vi "main.vi"() -> ()   [LabVIEW 2025]
uses:
  <vilib>/Handler Framework/CmdQueue/Enqueue Single.vi
  Classes/data log/data log.lvclass
  Classes/hardware/hardware.lvclass
  <vilib>/Handler Framework/Handler Framework.lvlib
panel:
  out "CMD Error":errorcluster
  out "x-y":dbl
  out "Waveform Chart":dbl(graph)
  out "Last Updated:":timestamp
  out "error out":errorcluster
  in  "save data":bool
  in  "Frequncy [Hz]":u16(slide)=1 max=10 step=1 scale=0.0..10.0
  in  "Reference Temperature [°F]":dbl(slide)=65.0 min=65.0 max=750.0 scale=0.0..500.0
  out "Temperatures:":dbl[](array[numeric]) format="%.1g"
  out "Duty Cycles:":dbl[](array[numeric]) format="%.1g"
  out "Relay Duty Cycle":T1(graph)
  out "Temperatures":T2(graph)
  in  "heat":bool
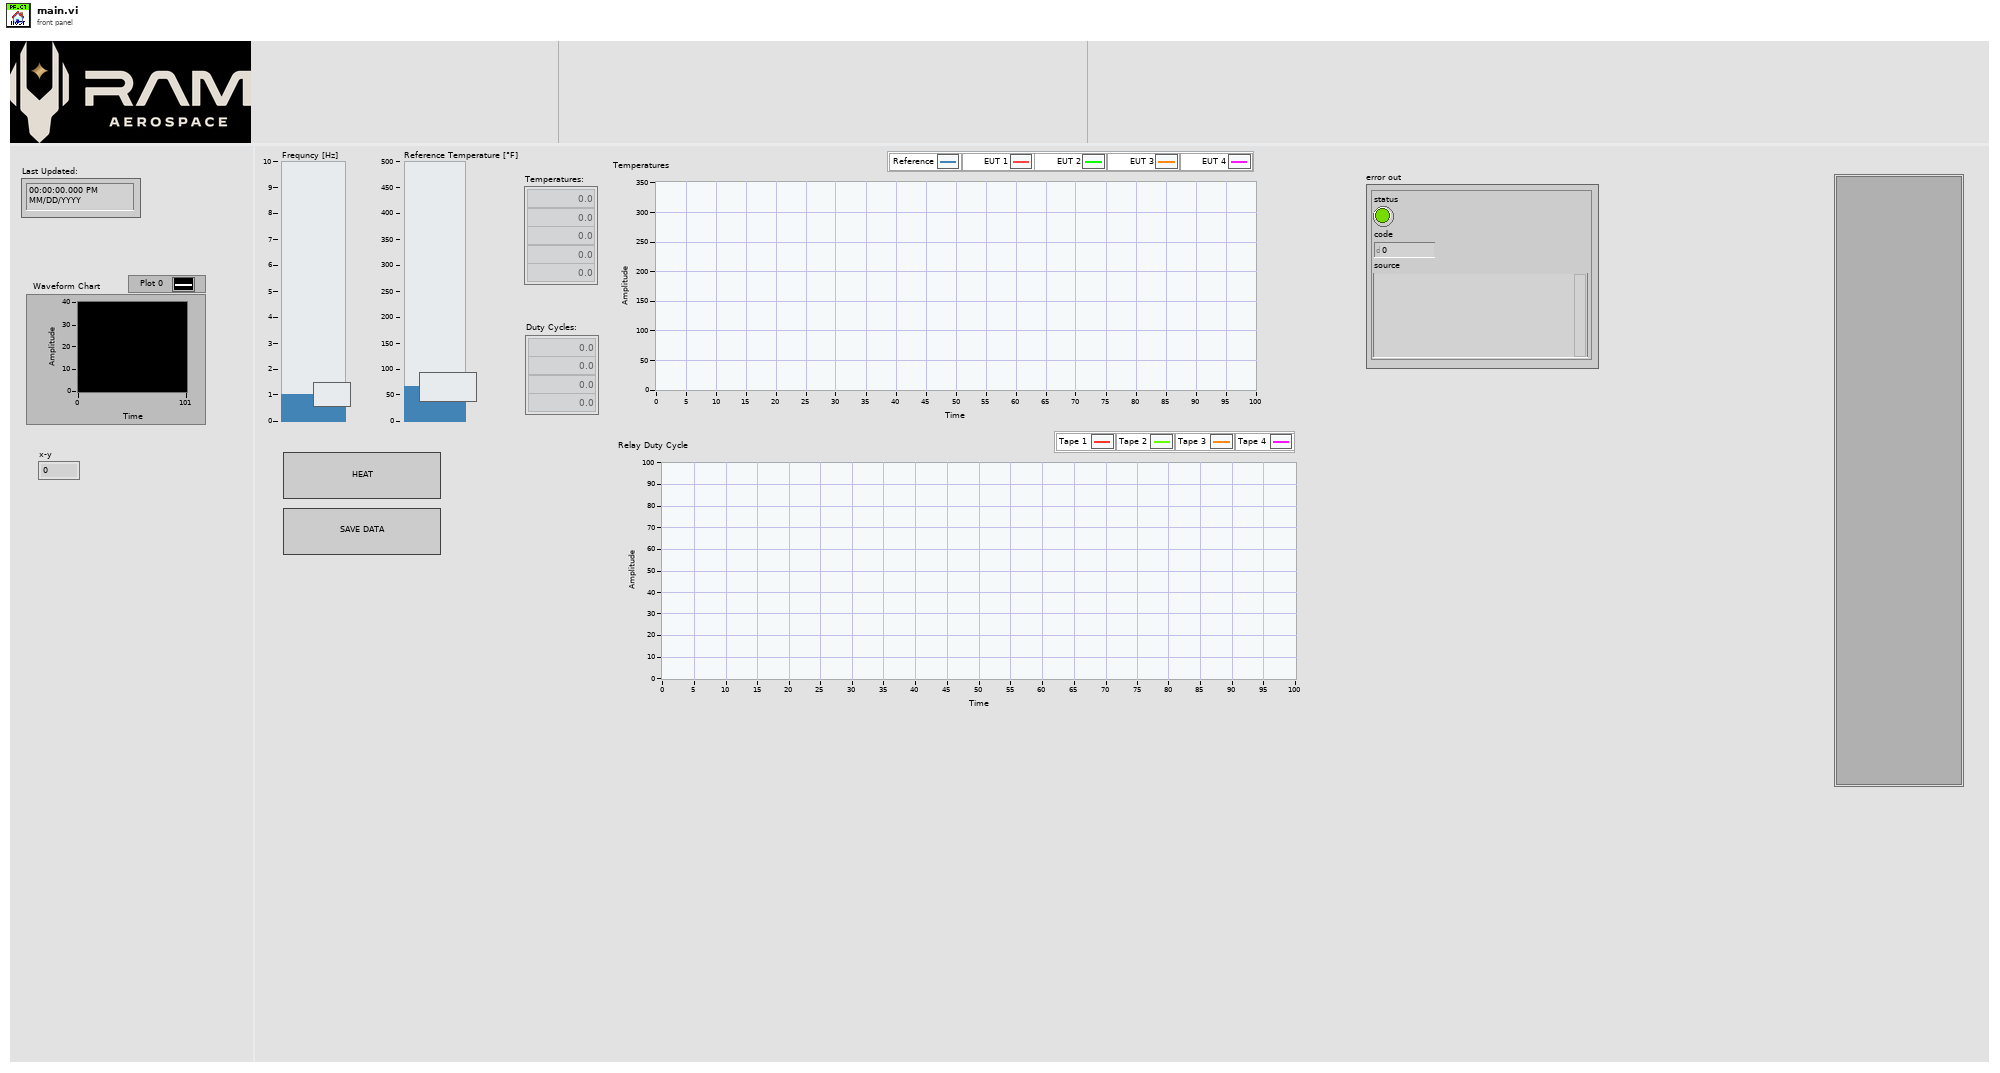
[diagram p1: front panel]
types:
  T1 = cluster{"Duty Cycle Array[0]":dbl, "Duty Cycle Array[1]":dbl, "Duty Cycle Array[2]":dbl, "Duty Cycle Array[3]":dbl, "Duty Cycle Array[4]":dbl, "Duty Cycle Array[5]":dbl, "Duty Cycle Array[6]":dbl, "Duty Cycle Array[7]":dbl, "Duty Cycle Array[8]":dbl}
  T2 = cluster{"Temperature Array[0]":dbl, "Temperature Array[1]":dbl, "Temperature Array[2]":dbl, "Temperature Array[3]":dbl, "Temperature Array[4]":dbl, "Temperature Array[5]":dbl, "Temperature Array[6]":dbl, "Temperature Array[7]":dbl, "Temperature Array[8]":dbl}
  T3 = cluster{"Tape 1":refnum<class "controller.lvclass">, "Tape 2":refnum<class "controller.lvclass">, "Tape 3":refnum<class "controller.lvclass">, "Tape 4":refnum<class "controller.lvclass">, "Hardware":refnum<class "hardware.lvclass">, "Data Log":refnum<class "data log.lvclass">}
  T4 = cluster{"[0]":dbl, "[1]":dbl, "[2]":dbl, "[3]":dbl, "[4]":dbl, "[5]":dbl, "[6]":dbl, "[7]":dbl, "[8]":dbl}
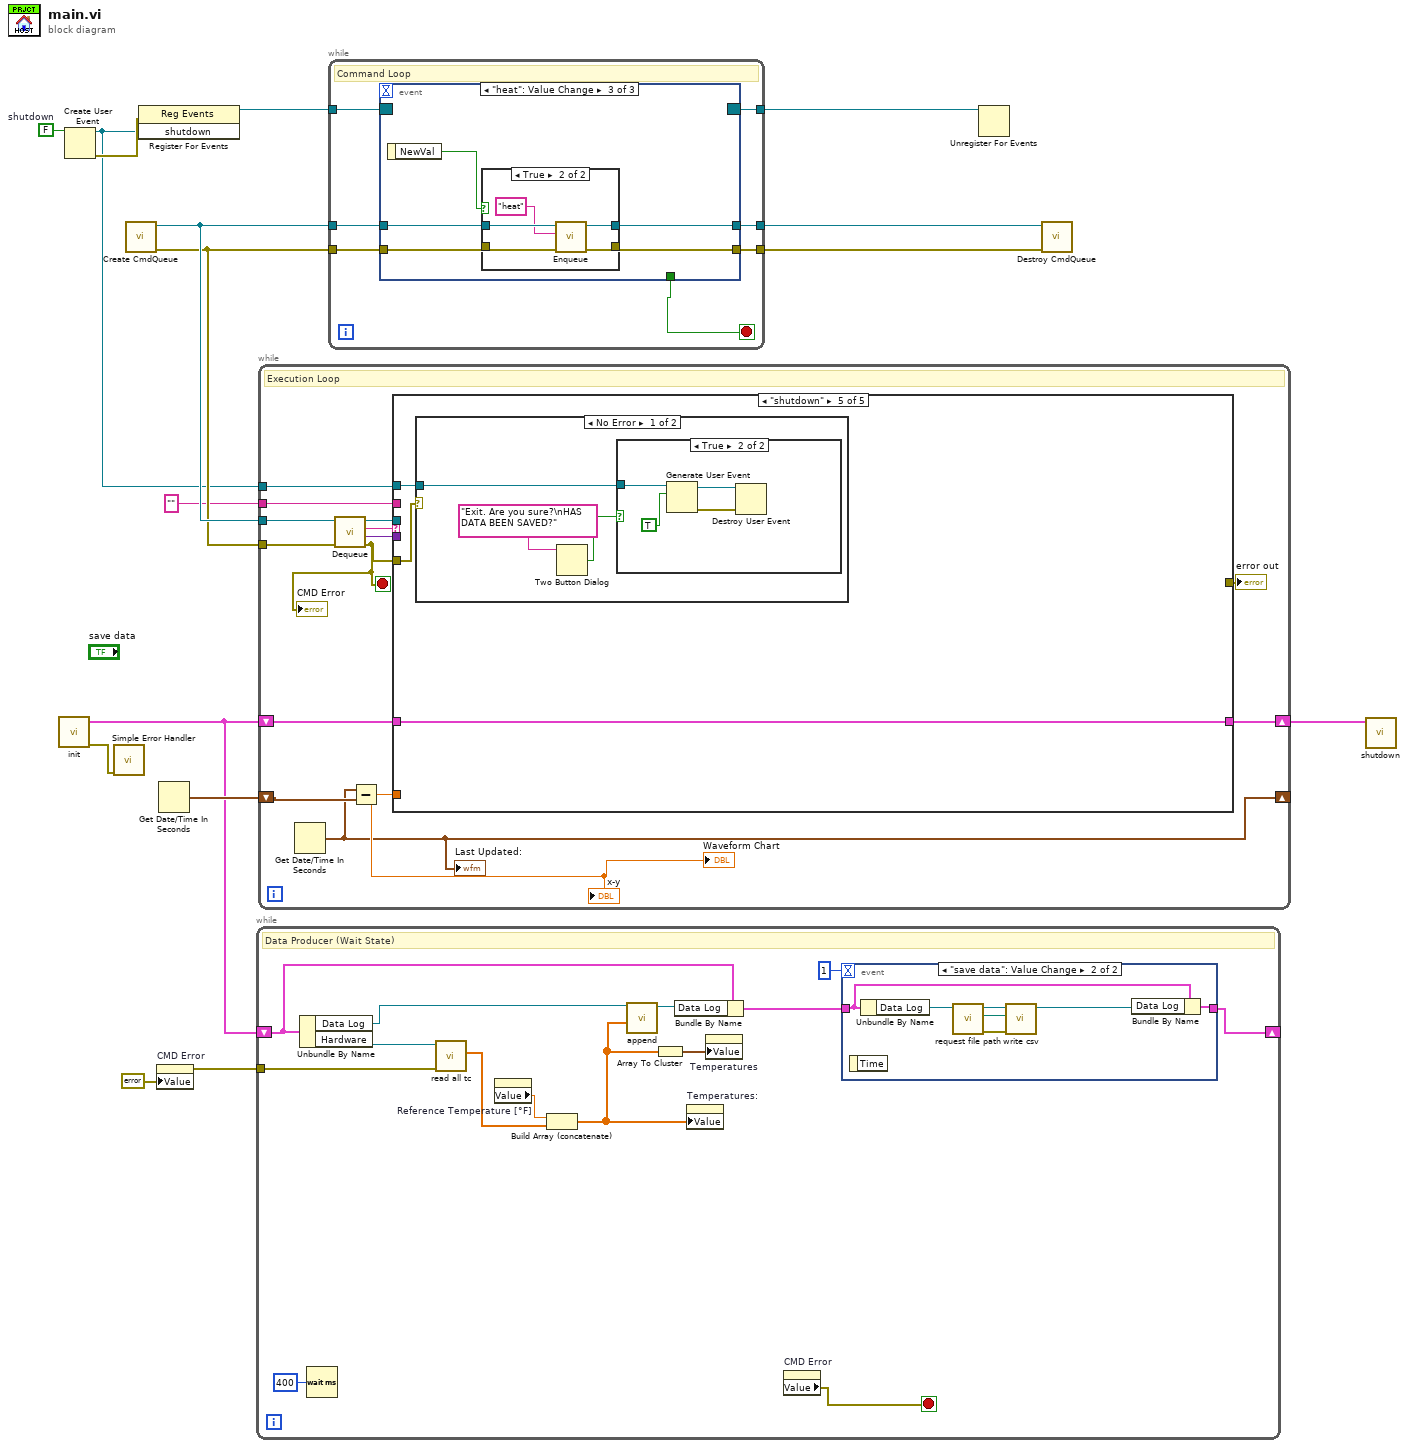
[diagram p0: block diagram]
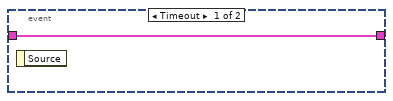
[diagram p2: hidden frame]
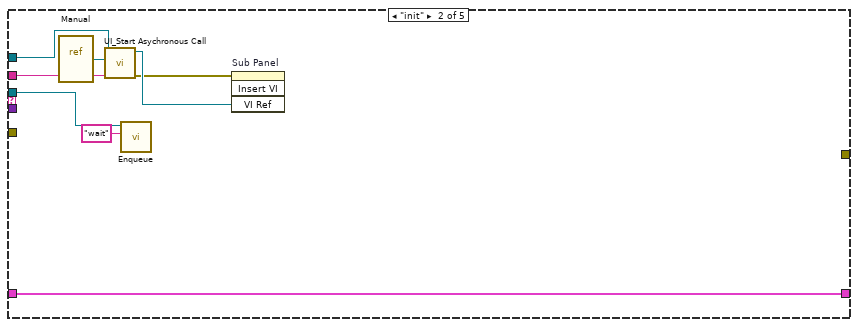
[diagram p4: hidden frame]
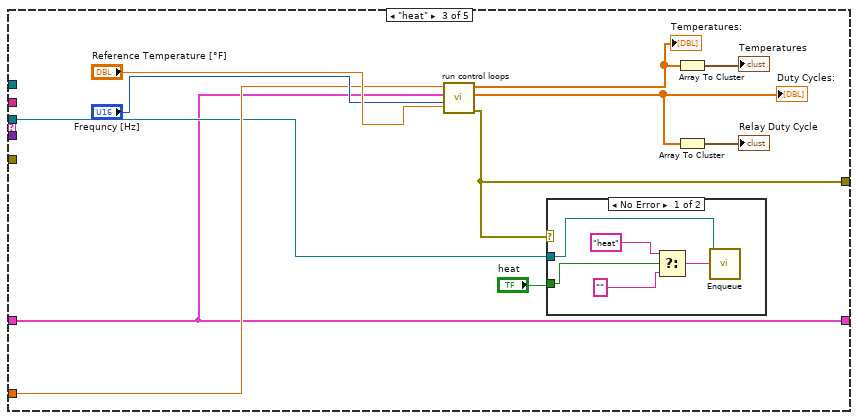
[diagram p5: hidden frame]
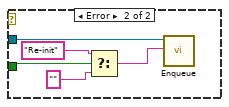
[diagram p6: hidden frame]
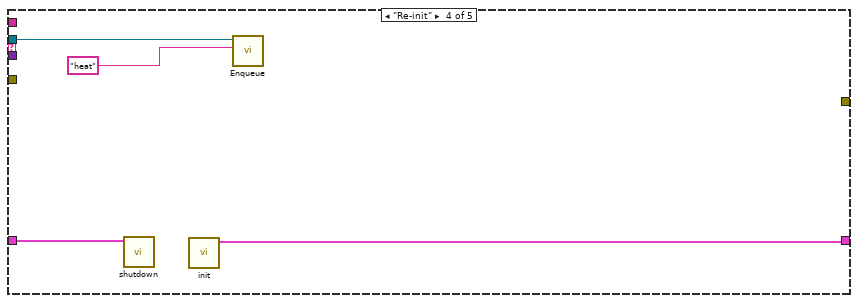
[diagram p7: hidden frame]
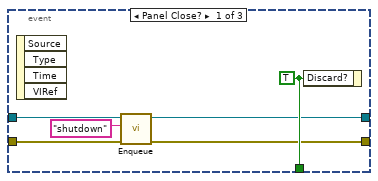
[diagram p10: hidden frame]
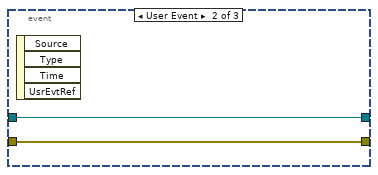
[diagram p11: hidden frame]
diagram:
  w12 = FALSE  # shutdown
  n1 = call "init.vi"() -> ("error"=w3:errorcluster, "input cluster"=w4:T3)  [unwired: 10 in]
  n2 = Create User Event(user event datatype=w12) -> (user event=w7:refnum<user-event>, error out=w8:errorcluster)  [unwired: 1 in]
  n3 = call <vilib>:"Simple Error Handler.vi"("error in (no error)"=w3) -> ()  [unwired: 4 in, 5 out]
  n4 = call <vilib>:"Create CmdQueue.vi"() -> ("error out"=w13:errorcluster, "CmdQueue out"=w14:refnum<queue>)  [unwired: 10 in]
  n5 = register-events(error in=w8, w7) -> (reference out=w11:refnum<event-registration>)  [unwired: 1 in, 1 out]
  n6 = property on="CMD Error" class="Clust (strict)"("Value"=errorcluster {"status"=FALSE, "code"=0, "source"=""} ("CMD Error")) -> (error out=w1:errorcluster)  [unwired: 2 in, 1 out]
  n7 = Get Date/Time In Seconds() -> (seconds since 1Jan1904=w5:timestamp)
  n8 = while {
    shift-right: [w17] -> _
    shift-left: w4 -> [w25]
    tunnel: w1 -> [w20]
    stop <- w21 stop-if-true
    # "Data Producer (Wait State)"
    n9 = Unbundle By Name(w25) -> ("Data Log"=w26:refnum<class "data log.lvclass">, "Hardware"=w29:refnum<class "hardware.lvclass">)
    n10 = Wait (ms)(milliseconds to wait=u32 400) -> ()  [unwired: 1 out]
    n11 = call-dynamic "read all tc.vi"("error in (no error)"=w20, "hardware in"=w29) -> ("Temperatures"=w24:dbl[])  [unwired: 7 in, 2 out]
    n12 = property on="Reference Temperature [°F]" class="Slide (strict)"() -> ("Value"=w23:dbl)  [unwired: 2 in, 2 out]
    n13 = Build Array (concatenate)(w23, w24) -> (w22:dbl[])
    n14 = call-dynamic "append.vi"("data"=w22, "data log in"=w26) -> ("data log out"=w28:refnum<class "data log.lvclass">)  [unwired: 8 in, 1 out]
    n15 = Array To Cluster(array=w22) -> (cluster=w27:T4)
    n16 = Bundle By Name(cluster=w25, "Data Log"=w28) -> (w18:T3)
    n17 = property on="Temperatures:" class="Arr (strict)"("Value"=w22) -> ()  [unwired: 2 in, 2 out]
    n18 = property on="Temperatures" class="WFChart (strict)"("Value"=w27) -> ()  [unwired: 2 in, 2 out]
    n19 = property on="CMD Error" class="Clust (strict)"() -> ("Value"=w21:errorcluster)  [unwired: 2 in, 2 out]
    n20 = event shown="[1] \"save data\": Value Change" {
      selector: _ -> [_ _]
      dyn-events: _ -> [_ _]
      timeout: 1 -> [_ _]
      tunnel: w18 -> [w31 w37]
      tunnel: [w31 w38] -> w17
      event Timeout {
        n21 = event-data() -> ()  [unwired: 1 in, 1 out]
      }
      event "save data": Value Change {
        n22 = event-data() -> ()  [unwired: 1 in, 1 out]
        n23 = Unbundle By Name(w37) -> ("Data Log"=w36:refnum<class "data log.lvclass">)
        n24 = call-dynamic "request file path.vi"("data log in"=w36) -> ("error out"=w35:errorcluster, "selected path"=w34:path, "data log out"=w33:refnum<class "data log.lvclass">)  [unwired: 8 in]
        n25 = call-dynamic "write csv.vi"("error in (no error)"=w35, "file path (dialog if empty)"=w34, "data log in"=w33) -> ("data log out"=w32:refnum<class "data log.lvclass">)  [unwired: 7 in, 1 out]
        n26 = Bundle By Name(cluster=w37, "Data Log"=w32) -> (w38:T3)
      }
    }
  }
  n27 = while {
    tunnel: w14 -> [w52]
    tunnel: w13 -> [w49]
    tunnel: w7 -> [w48]
    tunnel: "" ("String") -> [w47]
    shift-right: [w45] -> w6
    shift-left: w4 -> [w44]
    shift-right: [w40] -> _
    shift-left: w5 -> [w43]
    stop <- w46 stop-if-true
    # "Execution Loop"
    n28 = Get Date/Time In Seconds() -> (seconds since 1Jan1904=w40:timestamp)
    "Last Updated:" <- w40
    n29 = call <vilib>:"Dequeue.vi"("error in (no error)"=w49, "CmdQueue in"=w52) -> ("error out"=w46:errorcluster, "value"=w50:variant, "cmd"=w51:string, "CmdQueue out"=w42:refnum<queue>)  [unwired: 5 in, 1 out]
    "CMD Error" <- w46
    n30 = Subtract(x=w40, y=w43) -> (x-y=w41:dbl)
    "Waveform Chart" <- w41
    "x-y" <- w41
    n31 = case shown="\"shutdown\"" w51 {
      tunnel: w50 -> [_ _ _ _ _]
      tunnel: w48 -> [_ w58 _ _ w89]
      tunnel: w47 -> [_ w57 _ _ _]
      tunnel: w46 -> [_ _ _ _ w88]
      tunnel: w44 -> [w53 w56 w62 w86 w87]
      tunnel: [w53 w56 w62 w85 w87] -> w45
      tunnel: w41 -> [_ _ w70 _ _]
      tunnel: w42 -> [_ w55 w66 w84 _]
      tunnel: [_ _ w64 _ _] -> w39
      frame "False", Default {
      }
      frame "init" {
        n32 = vi-ref "Manual.vi"() -> (w61:refnum<vi>)
        n33 = call "UI_Start Asychronous Call.vi"("String"=w57, "VI Refnum"=w61, "User Event in"=w58) -> ("error out"=w59:errorcluster, "VI out"=w60:refnum<vi>)  [unwired: 7 in]
        n34 = call-poly <vilib>:"Enqueue.vi"("Command"="wait", "CmdQueue in"=w55) -> ()  [unwired: 8 in, 2 out]
        n35 = invoke on="Sub Panel" class="SubPnl" method="Insert VI"(error in=w59, "VI Ref"=w60) -> ()  [unwired: 2 in, 4 out]
      }
      frame "heat" {
        n36 = call "run control loops.vi"("Reference Temperature [°F]"="Reference Temperature [°F]", "Frequncy [Hz]"="Frequncy [Hz]", "input cluster"=w62, "dt [s]"=w70) -> ("error out"=w64:errorcluster, "Duty Cycle Array"=w68:dbl[], "Temperature Array"=w63:dbl[])  [unwired: 4 in, 1 out]
        "Duty Cycles:" <- w68
        "Temperatures:" <- w63
        n37 = case shown="No Error" w64 {
          tunnel: w66 -> [w76 w82]
          tunnel: "heat" -> [w75 w80]
          frame No Error {
            n38 = Select(t="heat", s=w75, f="") -> (s? t:f=w77:string)
            n39 = call-poly <vilib>:"Enqueue.vi"("Command"=w77, "CmdQueue in"=w76) -> ()  [unwired: 8 in, 2 out]
          }
          frame Error {
            n40 = Select(t="Re-init" ("Command"), s=w80, f="" ("t")) -> (s? t:f=w81:string)
            n41 = call-poly <vilib>:"Enqueue.vi"("Command"=w81, "CmdQueue in"=w82) -> ()  [unwired: 8 in, 2 out]
          }
        }
        n42 = Array To Cluster(array=w63) -> (cluster=→"Temperatures":T2)
        n43 = Array To Cluster(array=w68) -> (cluster=→"Relay Duty Cycle":T1)
      }
      frame "Re-init" {
        n44 = call "shutdown.vi"("input cluster"=w86) -> ()  [unwired: 11 in]
        n45 = call "init.vi"() -> ("input cluster"=w85:T3)  [unwired: 10 in, 1 out]
        n46 = call-poly <vilib>:"Enqueue.vi"("Command"="heat", "CmdQueue in"=w84) -> ()  [unwired: 8 in, 2 out]
      }
      frame "shutdown" {
        n47 = case shown="No Error" w88 {
          tunnel: w89 -> [w90 _]
          frame No Error {
            n48 = Two Button Dialog(message="Exit. Are you sure?\nHAS DATA BEEN SAVED?") -> (T button?=w91:bool)  [unwired: 2 in]
            n49 = case shown="True" w91 {
              tunnel: w90 -> [_ w96]
              frame False {
              }
              frame True {
                n50 = Generate User Event(user event=w96, event data cluster=TRUE ("event data")) -> (user event out=w94:refnum<user-event>, error out=w93:errorcluster)  [unwired: 2 in]
                n51 = Destroy User Event(user event=w94, error in=w93) -> ()  [unwired: 1 out]
              }
            }
          }
          frame Error {
          }
        }
      }
    }
    "error out" <- w39
  }
  n52 = while {
    tunnel: w14 -> [w101]
    tunnel: [w99] -> w16
    tunnel: w13 -> [w100]
    tunnel: [w98] -> w15
    tunnel: w11 -> [w103]
    tunnel: [w102] -> w10
    stop <- w97 stop-if-true
    # "Command Loop"
    n53 = event shown="[2] \"heat\": Value Change" {
      selector: w103 -> [_ _ _]
      dyn-events: [_ _ _] -> w102
      timeout: _ -> [_ _ _]
      tunnel: w101 -> [w108 w111 w113]
      tunnel: w100 -> [w107 w110 w114]
      tunnel: [w105 w111 w116] -> w99
      tunnel: [w104 w110 w115] -> w98
      tunnel: [w106 _ _] -> w97
      event Panel Close? {
        w106 = TRUE ("Discard?")
        n54 = event-data() -> ()  [unwired: 1 in, 4 out]
        n55 = call-poly <vilib>:"Enqueue.vi"("error in (no error)"=w107, "Command"="shutdown", "CmdQueue in"=w108) -> ("error out"=w104:errorcluster, "CmdQueue out"=w105:refnum<queue>)  [unwired: 7 in]
        n56 = event-data("Discard?"=w106) -> ()  [unwired: 1 in, 1 out]
      }
      event User Event {
        n57 = event-data() -> ()  [unwired: 1 in, 4 out]
      }
      event "heat": Value Change {
        n58 = event-data() -> ("NewVal"=w112:bool)  [unwired: 1 in]
        n59 = case shown="True" w112 {
          tunnel: [w118 w123] -> w116
          tunnel: [w117 w122] -> w115
          tunnel: w114 -> [w117 w121]
          tunnel: w113 -> [w118 w120]
          frame False {
          }
          frame True {
            n60 = call-poly <vilib>:"Enqueue.vi"("error in (no error)"=w121, "Command"="heat", "CmdQueue in"=w120) -> ("error out"=w122:errorcluster, "CmdQueue out"=w123:refnum<queue>)  [unwired: 7 in]
          }
        }
      }
    }
  }
  n61 = Unregister For Events(event registration refnum=w10) -> ()  [unwired: 1 in, 1 out]
  n62 = call <vilib>:"Destroy CmdQueue.vi"("error in (no error)"=w15, "CmdQueue in"=w16) -> ()  [unwired: 9 in, 1 out]
  n63 = call "shutdown.vi"("input cluster"=w6) -> ()  [unwired: 11 in]
